vi "Signal Page.vi"(8 "error in (no error)":errorcluster, 11 "Node Ptr":T1 format="%.0x") -> (0 "error out":errorcluster)   [LabVIEW 2023, in "J1939 Addon System Explorer.lvlib"]
uses:
  J1939 Addon System Explorer.lvlib
  <vilib>/NI VeriStand/Custom Device API/Custom Device Item Ref.ctl
  Addon Shared/SubVIs/Constants.vi
  <vilib>/NI VeriStand/Custom Device API/Custom Device API.lvlib
  Addon Shared/J1939 Addon Shared.lvlib
panel:
  in  "SHDocVw.IWebBrowser2":refnum<k7>(container)
  in  "Default Data":dbl
  in  "Header":cluster{"Section Name":string}={"Section Name"="Signal Settings"}
  in  "Description":string
  out "Name":string
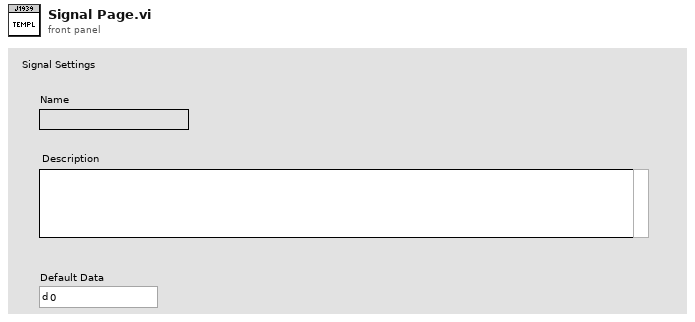
[diagram p1: front panel]
types:
  T1 = typedef "Custom Device API.lvlib/Custom Device Item Ref.ctl" = u64
  T2 = typedef "Custom Device API.lvlib/Custom Device Item Info.ctl" = cluster{"Name":string, "Is Channel":bool, "GUID":string, "Is Waveform":bool}
  T3 = typedef "Custom Device API.lvlib/Custom Device Channel.ctl" = cluster{"Type":T4, "Units":string, "Default Value":dbl, "Faultable":bool, "Scalable":bool}
  T4 = typedef "Custom Device API.lvlib/Custom Device Channel Type.ctl" = enum16{"Input", "Output"}
  T5 = typedef "Custom Device API.lvlib/Custom Device Commands.ctl" = enum16{"Default", "Item renamed", "Shutdown", "Dynamic button pressed"}
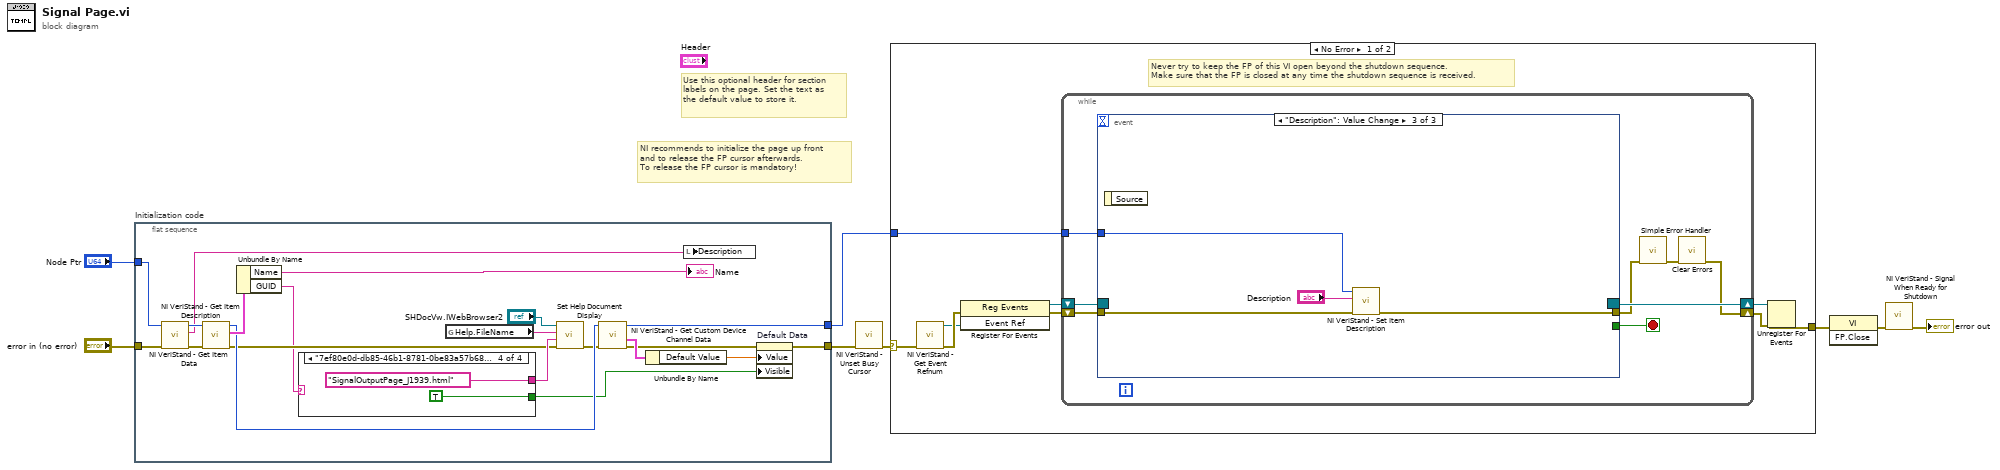
[diagram p0: block diagram]
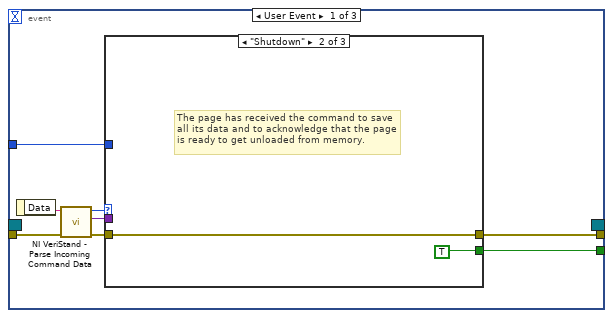
[diagram p2: hidden frame]
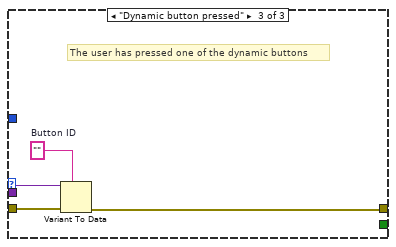
[diagram p4: hidden frame]
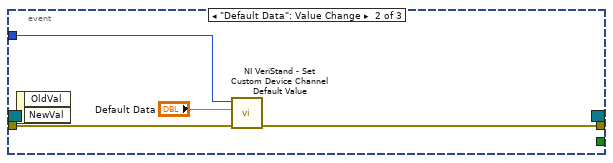
[diagram p5: hidden frame]
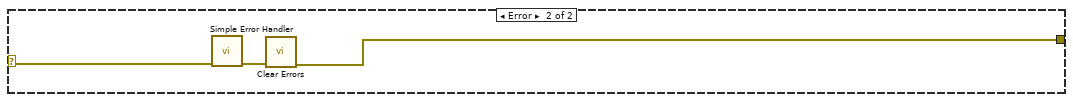
[diagram p6: hidden frame]
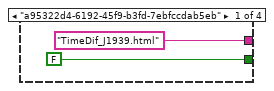
[diagram p7: hidden frame]
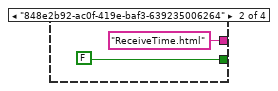
[diagram p8: hidden frame]
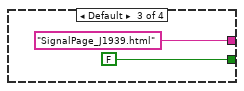
[diagram p9: hidden frame]
diagram:
  # "Use this optional header for section labels on the page. Set the text as the default value to store it."
  # "NI recommends to initialize the page up front\nand to release the FP cursor afterwards.\nTo release the FP cursor is mandatory!"
  n1 = flat-sequence "Initialization code" {
    tunnel: "error in (no error)" -> [w19]
    tunnel: "Node Ptr" -> [w27]
    tunnel: [w12] -> w4
    tunnel: [w22] -> w1
    frame #0 {
      n2 = call <vilib>:"NI VeriStand - Get Item Description.vi"("error in (no error)"=w19, "Item Ref in"=w27) -> ("error out"=w25:errorcluster, "Description"=w26:string, "Item Ref out"=w28:T1)  [unwired: 7 out]
      n3 = call <vilib>:"NI VeriStand - Get Item Data.vi"("error in (no error)"=w25, "Item Ref in"=w28) -> ("error out"=w15:errorcluster, "Item Info"=w24:T2, "Item Ref out"=w23:T1)  [unwired: 7 out]
      n4 = Unbundle By Name(w24) -> ("Name"=→"Name":string, "GUID"=w14:string)
      n5 = case shown="\"7ef80e0d-db85-46b1-8781-0be83a57b682\"" w14 {
        tunnel: ["TimeDif_J1939.html" ("HTML File") "ReceiveTime.html" ("HTML File") "SignalPage_J1939.html" ("HTML File") "SignalOutputPage_J1939.html" ("HTML File")] -> w16
        tunnel: [FALSE FALSE FALSE TRUE] -> w10
        frame "a95322d4-6192-45f9-b3fd-7ebfccdab5eb" {
        }
        frame "848e2b92-ac0f-419e-baf3-639235006264" {
        }
        frame Default {
        }
        frame "7ef80e0d-db85-46b1-8781-0be83a57b682" {
        }
      }
      n6 = global read "Constants.vi" "Help.FileName"() -> (w9:string)
      n7 = call "Set Help Document Display.vi"("error in (no error)"=w15, "HTML File"=w16, "Main CHM File"=w9, "SHDocVw.IWebBrowser2"="SHDocVw.IWebBrowser2") -> ("error out"=w17:errorcluster)  [unwired: 7 in]
      n8 = call <vilib>:"NI VeriStand - Get Custom Device Channel Data.vi"("error in (no error)"=w17, "Channel Ref in"=w23) -> ("error out"=w13:errorcluster, "Channel"=w21:T3, "Channel Ref out"=w22:T1)  [unwired: 4 in, 3 out]
      n9 = Unbundle By Name(w21) -> ("Default Value"=w11:dbl)
      n10 = local write "Description"(w26) -> ()
      n11 = property on="Default Data" class="DigNum (strict)"(error in=w13, "Value"=w11, "Visible"=w10) -> (error out=w12:errorcluster)  [unwired: 1 in, 1 out]
    }
  }
  n12 = call <vilib>:"NI VeriStand - Unset Busy Cursor.vi"("error in (no error)"=w4) -> ("error out"=w3:errorcluster)  [unwired: 10 out]
  n13 = case shown="No Error" w3 {
    selector: w3 -> [w37 w79]
    tunnel: [w42 w77] -> w8
    tunnel: w1 -> [w38 _]
    frame No Error {
      # "Never try to keep the FP of this VI open beyond the shutdown sequence.\nMake sure that the FP is closed at any time the shutdown sequence is received."
      n14 = call <vilib>:"NI VeriStand - Get Event Refnum.vi"("error in (no error)"=w37) -> ("error out"=w45:errorcluster, "Event Ref"=w41:refnum<user-event>)  [unwired: 9 out]
      n15 = register-events(error in=w45, w41) -> (reference out=w39:refnum<event-registration>, error out=w40:errorcluster)  [unwired: 1 in]
      n16 = while {
        tunnel: w38 -> [w49]
        shift-right: [w46] -> w43
        shift-left: w40 -> [w52]
        shift-right: [w53] -> w44
        shift-left: w39 -> [w51]
        stop <- w50 stop-if-true
        n17 = event shown="[2] \"Description\": Value Change" {
          selector: w51 -> [_ _ _]
          dyn-events: [_ _ _] -> w53
          timeout: _ -> [_ _ _]
          tunnel: w52 -> [w61 w70 w75]
          tunnel: [w57 _ _] -> w50
          tunnel: [w56 w69 w74] -> w48
          tunnel: w49 -> [w55 w72 w76]
          event User Event {
            n18 = event-data() -> ("Data"=w60:string)  [unwired: 1 out]
            n19 = call <vilib>:"NI VeriStand - Parse Incoming Command Data.vi"("error in (no error)"=w61, "Incoming data"=w60) -> ("error out"=w59:errorcluster, "Outgoing data"=w54:variant, "Action"=w58:T5)  [unwired: 7 out]
            n20 = case shown="\"Shutdown\"" w58 {
              tunnel: w59 -> [w62 w63 w68]
              tunnel: [_ TRUE _] -> w57
              tunnel: [w62 w63 w65] -> w56
              tunnel: w55 -> [_ _ _]
              tunnel: w54 -> [_ _ w67]
              frame "Default", Default {
              }
              frame "Shutdown" {
                # "The page has received the command to save all its data and to acknowledge that the page is ready to get unloaded from memory."
              }
              frame "Dynamic button pressed" {
                w66 = ""  # Button ID
                # "The user has pressed one of the dynamic buttons"
                n21 = Variant To Data(error in=w68, type=w66, Variant=w67) -> (error out=w65:errorcluster)  [unwired: 1 out]
              }
            }
          }
          event "Default Data": Value Change {
            n22 = event-data() -> ()  [unwired: 3 out]
            n23 = call <vilib>:"NI VeriStand - Set Custom Device Channel Default Value.vi"("error in (no error)"=w70, "Default Value"="Default Data", "Channel Ref in"=w72) -> ("error out"=w69:errorcluster)  [unwired: 7 in, 1 out]
          }
          event "Description": Value Change {
            n24 = event-data() -> ()  [unwired: 2 out]
            n25 = call <vilib>:"NI VeriStand - Set Item Description.vi"("error in (no error)"=w75, "Description"="Description", "Item Ref in"=w76) -> ("error out"=w74:errorcluster)  [unwired: 8 out]
          }
        }
        n26 = call <vilib>:"Simple Error Handler.vi"("error in (no error)"=w48) -> ("error out"=w47:errorcluster)  [unwired: 1 in, 7 out]
        n27 = call <vilib>:"Clear Errors.vi"("error in (no error)"=w47) -> ("error out"=w46:errorcluster)  [unwired: 1 in, 5 out]
      }
      n28 = Unregister For Events(event registration refnum=w44, error in=w43) -> (error out=w42:errorcluster)
    }
    frame Error {
      n29 = call <vilib>:"Simple Error Handler.vi"("error in (no error)"=w79) -> ("error out"=w78:errorcluster)  [unwired: 1 in, 7 out]
      n30 = call <vilib>:"Clear Errors.vi"("error in (no error)"=w78) -> ("error out"=w77:errorcluster)  [unwired: 1 in, 5 out]
    }
  }
  n31 = invoke class="VI" method="FP.Close"(error in=w8) -> (error out=w7:errorcluster)  [unwired: 2 in, 2 out]
  n32 = call <vilib>:"NI VeriStand - Signal When Ready for Shutdown.vi"("error in (no error)"=w7) -> ("error out"=→"error out":errorcluster)  [unwired: 10 out]
